vi "Export.vi"(8 "error in":errorcluster, 11 "Objects":T1) -> (0 "error out":errorcluster)   [LabVIEW 2015, in "Modbus Module editor node.lvclass"]
uses:
  Modbus Module editor node.lvclass
  <vilib>/NI/DCAF/Tag Editor Core/Table API/Table Manager/object ref.ctl
  <vilib>/NI/DCAF/Tag Editor Core/Configuration Editor/Classes/Engine Parent/Engine Parent Editor Node.lvclass
  <vilib>/NI/DCAF/Tag Editor Core/Configuration Editor/Classes/Module editor node/module editor node.lvclass
  <vilib>/NI/DCAF/Tag Editor Core/Table API/Table Manager/Table Manager.lvclass
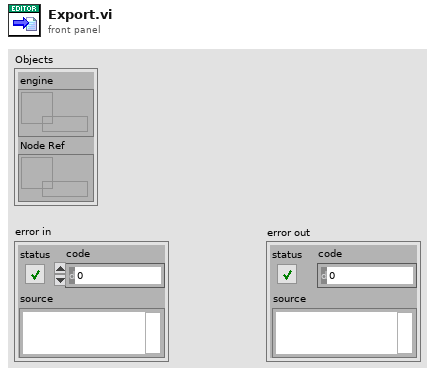
[diagram p1: front panel]
types:
  T1 = typedef "Table Manager.lvlib/Table Manager.lvclass/object ref.ctl" = cluster{"engine":refnum<data-value>, "Node Ref":refnum<data-value>}
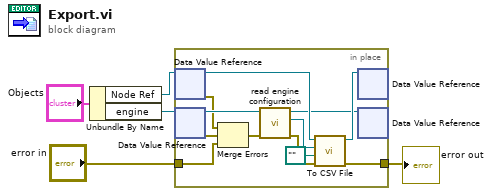
[diagram p0: block diagram]
diagram:
  n1 = Unbundle By Name("Objects") -> ("Node Ref"=w5:refnum<data-value>, "engine"=w4:refnum<data-value>)
  n2 = in-place {
    in-place-border: "error in" -> [w10]
    in-place-border: [w7] -> w1
    n3 = in-place-dvr #1(w5) -> (w17:refnum<class "module editor node.lvclass">, w12:errorcluster)
    n4 = in-place-dvr #2(w4) -> (w15:refnum<class "Engine Parent Editor Node.lvclass">, w11:errorcluster)
    n5 = Merge Errors(w12, w11, w10) -> (w9:errorcluster)
    n6 = call <vilib>:"read engine configuration.vi"("error in"=w9, "Engine Parent Editor Node in"=w15) -> ("error out"=w8:errorcluster, "engine configuration"=w14:refnum<class "engine configuration.lvclass">, "Engine Parent Editor Node out"=w13:refnum<class "Engine Parent Editor Node.lvclass">)  [unwired: 7 in]
    n7 = call-dynamic "To CSV File.vi"("error in (no error)"=w8, "Path"=path "", "engine configuration"=w14, "module editor node in"=w17) -> ("error out"=w7:errorcluster, "module editor node out"=w16:refnum<class "module editor node.lvclass">)  [unwired: 6 in]
    n8 = in-place-dvr #1(w16) -> ()  [unwired: 2 out]
    n9 = in-place-dvr #2(w13) -> ()  [unwired: 2 out]
  }
  "error out" <- w1
